vi "Get LV Color.vi"(8 "error in (no error)":errorcluster, 11 "CMY Color.lvclass in":refnum<class "CMY Color.lvclass">) -> (0 "error out":errorcluster, 2 "Color":u32(colorbox), 3 "CMY Color.lvclass out":refnum<class "CMY Color.lvclass">)   [LabVIEW 2020, in "CMY Color.lvclass"]
doc: "A method to get the LabVIEW color value corresponding the current color."
uses:
  CMY Color.lvclass
  CMY Color.lvclass/CMY Color.ctl
panel:
  # "expressionflow.com"
  # "Copyright (c) 2008 Tomi Maila. All rights reserved."
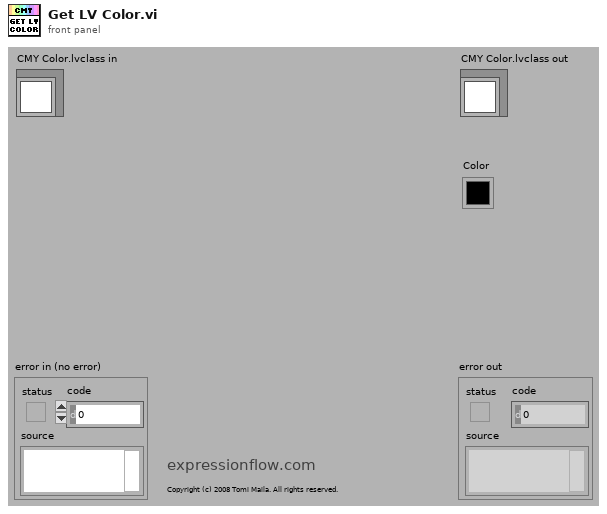
[diagram p1: front panel]
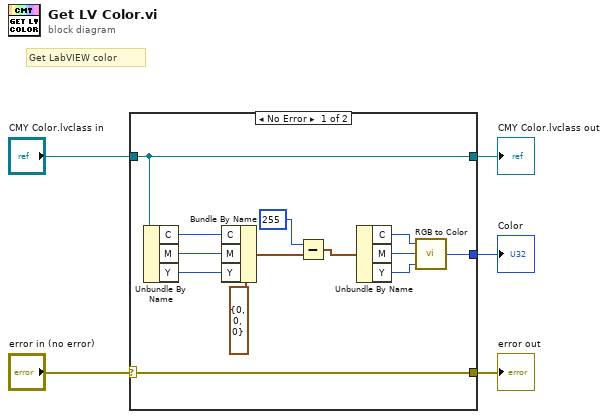
[diagram p0: block diagram]
diagram:
  # "Get LabVIEW color"
  n1 = case shown="No Error" "error in (no error)" {
    selector: "error in (no error)" -> [w18 w19]
    tunnel: [w18 w19] -> w4
    tunnel: "CMY Color.lvclass in" -> [w17 w20]
    tunnel: [w17 w20] -> w2
    tunnel: [w6 _] -> w1
    frame No Error {
      n2 = Unbundle By Name(w17) -> ("C"=w15:u8, "M"=w14:u8, "Y"=w13:u8)
      n3 = Bundle By Name(cluster=cluster{"C":u8, "M":u8, "Y":u8} {"C"=0, "M"=0, "Y"=0} ("RGB Value"), "C"=w15, "M"=w14, "Y"=w13) -> (w11:cluster{"C":u8, "M":u8, "Y":u8})
      n4 = Subtract(x=u8 255, y=w11) -> (x-y=w10:cluster{"C":u8, "M":u8, "Y":u8})
      n5 = Unbundle By Name(w10) -> ("C"=w8:u8, "M"=w9:u8, "Y"=w7:u8)
      n6 = call <vilib>:"RGB to Color.vi"("B"=w7, "G"=w9, "R"=w8) -> ("Color"=w6:u32)
    }
    frame Error {
    }
  }
  "error out" <- w4
  "CMY Color.lvclass out" <- w2
  "Color" <- w1
